vi "CC Convert DEC to String.vi"(8 "error in (no error)":errorcluster, 11 "DEC":dbl) -> (0 "error out":errorcluster, 2 "Declination":T1 {"Arc Sec" format="%0#2_6g"}, 3 "DEC String":string)   [LabVIEW 2024]
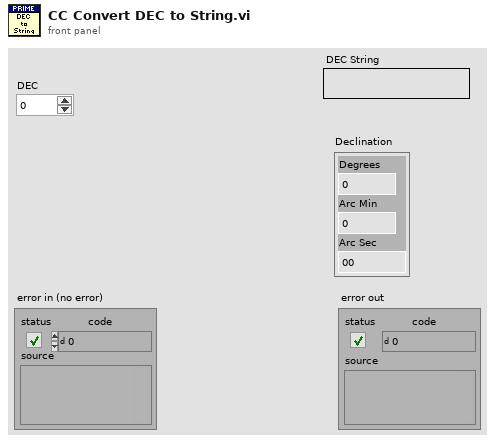
[diagram p1: front panel]
types:
  T1 = cluster{"Degrees":dbl, "Arc Min":dbl, "Arc Sec":dbl}
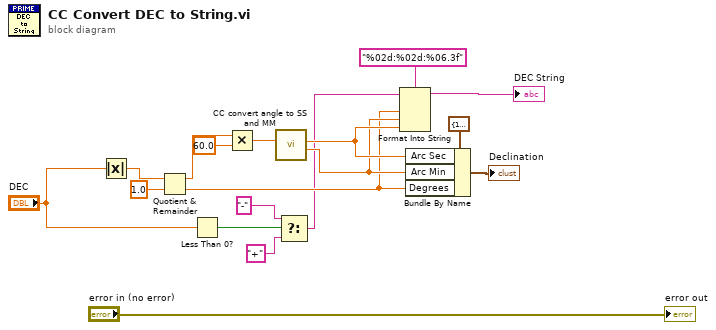
[diagram p0: block diagram]
diagram:
  n1 = Absolute Value(x="DEC") -> (abs(x)=w10:dbl)
  n2 = Quotient & Remainder(x=w10, y=1.0) -> (x-y*floor(x/y)=w16:dbl, floor(x/y)=w4:dbl)
  n3 = Less Than 0?(x="DEC") -> (x < 0?=w9:bool)
  n4 = Multiply(x=w16, y=60.0) -> (x*y=w7:dbl)
  n5 = call "CC convert angle to SS and MM.vi"("Angle"=w7) -> ("Minutes"=w5:dbl, "Seconds"=w6:dbl)  [unwired: 9 in]
  n6 = Select(t="-", s=w9, f="+") -> (s? t:f=w1:string)
  n7 = Format Into String(format string="%02d:%02d:%06.3f", initial string=w1, w4, w5, w6) -> (resulting string=→"DEC String":string)  [unwired: 1 in, 1 out]
  n8 = Bundle By Name(cluster=T1 {"Degrees"=10.0, "Arc Min"=2.0, "Arc Sec"=11.040000000001555} ("Declination"), "Arc Sec"=w6, "Arc Min"=w5, "Degrees"=w4) -> (→"Declination":T1)
  "error out" <- "error in (no error)"
